vi "Vision RIO Read Time.vi"() -> (3 "Rio Talking":bool)   [LabVIEW 2025]
uses:
  <vilib>/Rock Robotics/Network Tables/NT Read Number.vi
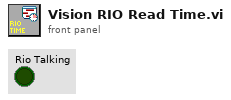
[diagram p1: front panel]
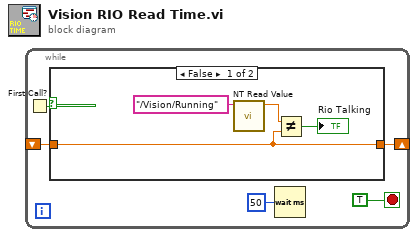
[diagram p0: block diagram]
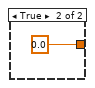
[diagram p2: hidden frame]
diagram:
  n1 = while {
    shift-right: [w4] -> _
    shift-left: _ -> [w3]
    stop <- TRUE stop-if-true
    n2 = First Call?() -> (First Call?: T/F=w5:bool)
    n3 = case shown="False" w5 {
      tunnel: [w8 0.0] -> w4
      tunnel: w3 -> [w8 _]
      frame False {
        n4 = call-poly <vilib>:"NT Read Value.vi"("name"="/Vision/Running" ("Name")) -> ("value"=w6:dbl)  [unwired: 8 in, 2 out]
        n5 = Not Equal?(x=w6, y=w8) -> (x != y?=→"Rio Talking":bool)
      }
      frame True {
      }
    }
    n6 = Wait (ms)(milliseconds to wait=u32 50) -> ()  [unwired: 1 out]
  }
